vi "AdvancedComparisonFunctions2.vi"() -> ()   [LabVIEW 2020]
panel:
  in  "x 2":dbl
  out "sqrt(x)":dbl
  out "min(x,y)":dbl
  out "max(x,y)":dbl
  in  "y":dbl
  in  "x":dbl
  out "s? t:f 2":string
  out "s? t:f":dbl
  in  "s":bool
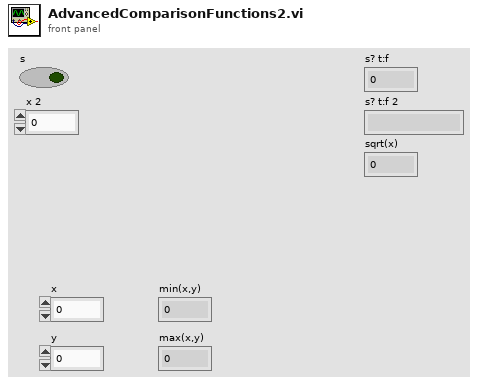
[diagram p1: front panel]
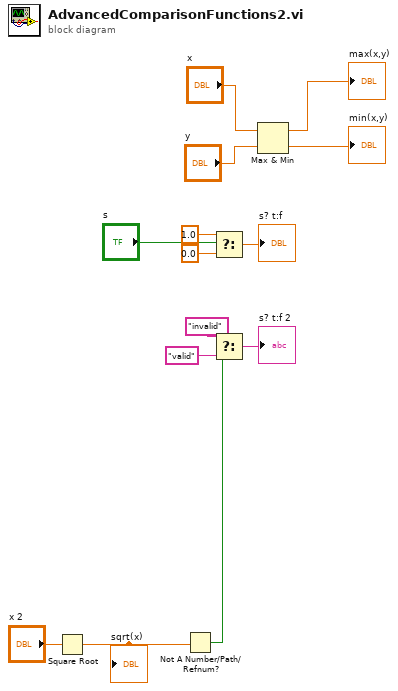
[diagram p0: block diagram]
diagram:
  n1 = Square Root(x="x 2") -> (sqrt(x)=w2:dbl)
  "sqrt(x)" <- w2
  n2 = Not A Number/Path/Refnum?(number/path/refnum=w2) -> (NaN/Path/Refnum?=w3:bool)
  n3 = Select(t=1.0, s="s", f=0.0) -> (s? t:f=→"s? t:f":dbl)
  n4 = Select(t="invalid", s=w3, f="valid") -> (s? t:f=→"s? t:f 2":string)
  n5 = Max & Min(x="x", y="y") -> (max(x,y)=→"max(x,y)":dbl, min(x,y)=→"min(x,y)":dbl)
